vi "TP059851_SimYokeShin_Quiz2B.vi"() -> ()   [LabVIEW 2020]
panel:
  out "Timer 2":dbl
  out "Green  2":bool
  out "Yellow   2":bool
  out "Red  2":bool
  out "Timer":dbl
  out "Green":bool
  out "Yellow":bool
  out "Red":bool
  # "A"
  # "B"
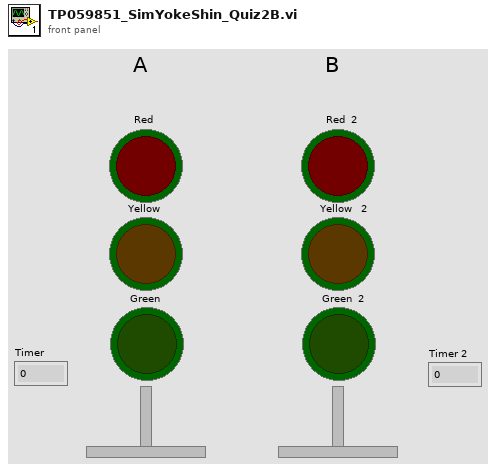
[diagram p1: front panel]
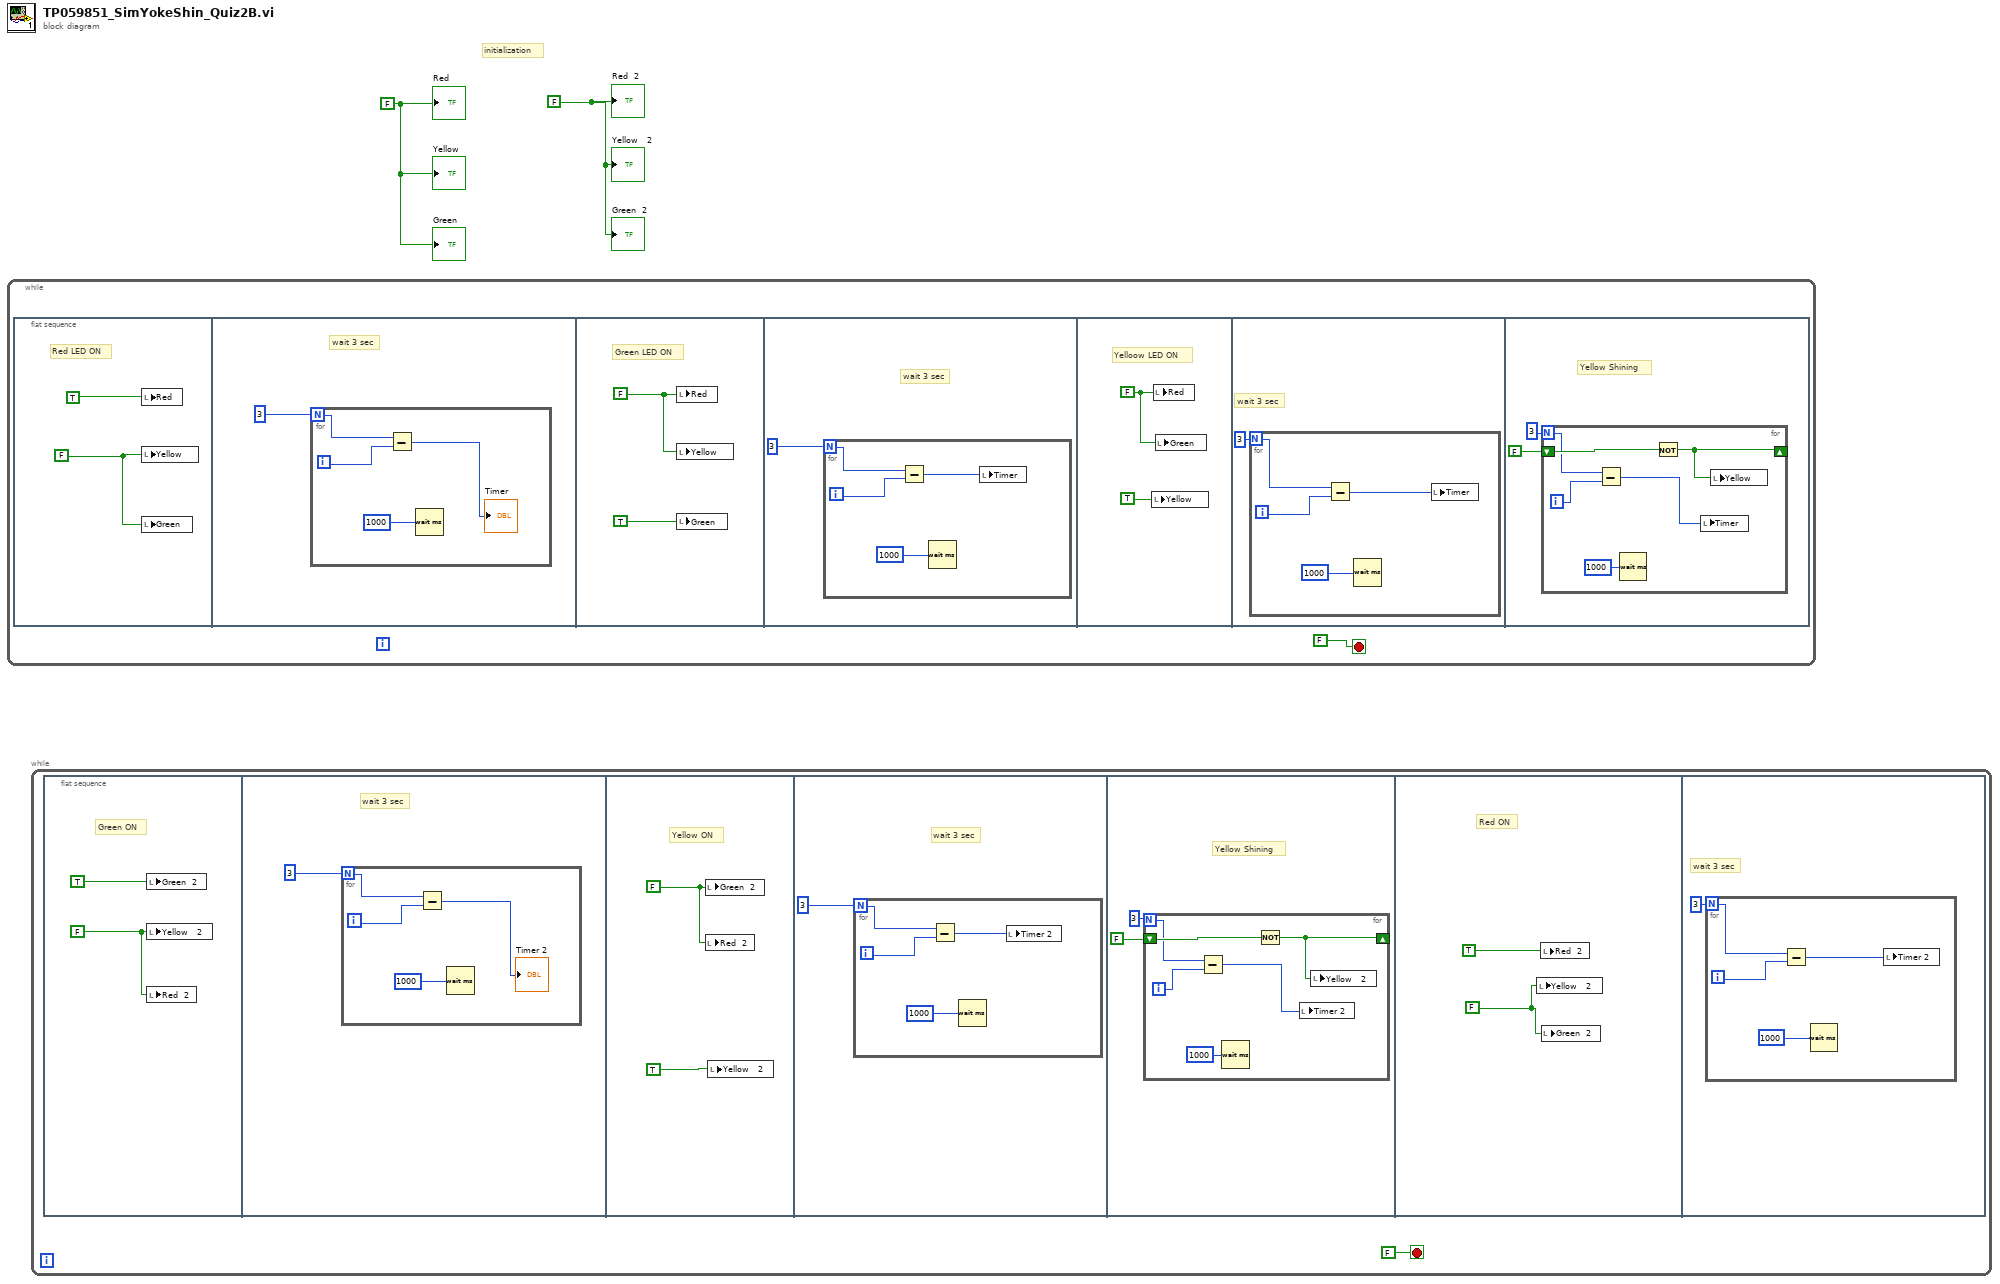
[diagram p0: block diagram]
diagram:
  w1 = FALSE ("Red  2")
  w2 = FALSE
  # "initialization"
  n1 = while {
    stop <- FALSE stop-if-true
    n2 = flat-sequence {
      frame #0 {
        w4 = FALSE
        # "Red LED ON"
        n3 = local write "Red"(TRUE) -> ()
        n4 = local write "Yellow"(w4) -> ()
        n5 = local write "Green"(w4) -> ()
      }
      frame #1 {
        # "wait 3 sec"
        n6 = for {
          N: u32 3 ("milliseconds to wait") -> [w10]
          i -> [w7]
          n7 = Subtract(x=w10, y=w7) -> (x-y=→"Timer":i32)
          n8 = Wait (ms)(milliseconds to wait=u32 1000) -> ()  [unwired: 1 out]
        }
      }
      frame #2 {
        w12 = FALSE ("Red LED")
        # "Green LED ON"
        n9 = local write "Red"(w12) -> ()
        n10 = local write "Yellow"(w12) -> ()
        n11 = local write "Green"(TRUE ("Green LED")) -> ()
      }
      frame #3 {
        # "wait 3 sec"
        n12 = for {
          N: u32 3 ("milliseconds to wait") -> [w17]
          i -> [w14]
          n13 = Subtract(x=w17, y=w14) -> (x-y=w15:i32)
          n14 = Wait (ms)(milliseconds to wait=u32 1000) -> ()  [unwired: 1 out]
          n15 = local write "Timer"(w15) -> ()
        }
      }
      frame #4 {
        w18 = FALSE ("Red LED")
        # "Yelloow LED ON"
        n16 = local write "Yellow"(TRUE ("Yellow LED")) -> ()
        n17 = local write "Red"(w18) -> ()
        n18 = local write "Green"(w18) -> ()
      }
      frame #5 {
        # "wait 3 sec"
        n19 = for {
          N: 3 -> [w24]
          i -> [w21]
          n20 = Subtract(x=w24, y=w21) -> (x-y=w22:i32)
          n21 = Wait (ms)(milliseconds to wait=u32 1000) -> ()  [unwired: 1 out]
          n22 = local write "Timer"(w22) -> ()
        }
      }
      frame #6 {
        # "Yellow Shining"
        n23 = for {
          N: 3 -> [w28]
          shift-right: [w30] -> _
          shift-left: FALSE -> [w32]
          i -> [w27]
          n24 = Subtract(x=w28, y=w27) -> (x-y=w29:i32)
          n25 = Wait (ms)(milliseconds to wait=u32 1000) -> ()  [unwired: 1 out]
          n26 = Not(x=w32) -> (.not. x?=w30:bool)
          n27 = local write "Timer"(w29) -> ()
          n28 = local write "Yellow"(w30) -> ()
        }
      }
    }
  }
  n29 = while {
    stop <- FALSE stop-if-true
    n30 = flat-sequence {
      frame #0 {
        w34 = FALSE ("Yellow   2")
        # "Green ON"
        n31 = local write "Green  2"(TRUE ("Green  2")) -> ()
        n32 = local write "Yellow   2"(w34) -> ()
        n33 = local write "Red  2"(w34) -> ()
      }
      frame #1 {
        # "wait 3 sec"
        n34 = for {
          N: u32 3 ("milliseconds to wait") -> [w40]
          i -> [w37]
          n35 = Subtract(x=w40, y=w37) -> (x-y=→"Timer 2":i32)
          n36 = Wait (ms)(milliseconds to wait=u32 1000) -> ()  [unwired: 1 out]
        }
      }
      frame #2 {
        w42 = FALSE ("Green  2")
        # "Yellow ON"
        n37 = local write "Green  2"(w42) -> ()
        n38 = local write "Red  2"(w42) -> ()
        n39 = local write "Yellow   2"(TRUE ("Yellow   2")) -> ()
      }
      frame #3 {
        # "wait 3 sec"
        n40 = for {
          N: u32 3 ("milliseconds to wait") -> [w47]
          i -> [w44]
          n41 = Subtract(x=w47, y=w44) -> (x-y=w45:i32)
          n42 = Wait (ms)(milliseconds to wait=u32 1000) -> ()  [unwired: 1 out]
          n43 = local write "Timer 2"(w45) -> ()
        }
      }
      frame #4 {
        # "Yellow Shining"
        n44 = for {
          N: 3 -> [w52]
          shift-right: [w50] -> _
          shift-left: FALSE -> [w55]
          i -> [w51]
          n45 = Subtract(x=w52, y=w51) -> (x-y=w53:i32)
          n46 = Wait (ms)(milliseconds to wait=u32 1000) -> ()  [unwired: 1 out]
          n47 = Not(x=w55) -> (.not. x?=w50:bool)
          n48 = local write "Timer 2"(w53) -> ()
          n49 = local write "Yellow   2"(w50) -> ()
        }
      }
      frame #5 {
        w56 = FALSE ("Yellow   2")
        # "Red ON"
        n50 = local write "Yellow   2"(w56) -> ()
        n51 = local write "Red  2"(TRUE ("Red  2")) -> ()
        n52 = local write "Green  2"(w56) -> ()
      }
      frame #6 {
        # "wait 3 sec"
        n53 = for {
          N: 3 -> [w62]
          i -> [w59]
          n54 = Subtract(x=w62, y=w59) -> (x-y=w60:i32)
          n55 = Wait (ms)(milliseconds to wait=u32 1000) -> ()  [unwired: 1 out]
          n56 = local write "Timer 2"(w60) -> ()
        }
      }
    }
  }
  "Red" <- w2
  "Yellow" <- w2
  "Green" <- w2
  "Yellow   2" <- w1
  "Green  2" <- w1
  "Red  2" <- w1
